vi "StopSpecificModules.vi"(8 "ErrorArray 2":errorcluster[](array[cluster]), 9 "ModuleList":string[](array[string]), 10 "ModuleIDs":i32[](array[numeric])=[-1, -1, -1], 11 "Test.lvclass 2":refnum<class "Test.lvclass">) -> (0 "ErrorArray":errorcluster[](array[cluster]), 3 "Test.lvclass":refnum<class "Test.lvclass">)   [LabVIEW 2018, in "Test.lvclass"]
uses:
  Test.lvclass
  Test.lvclass/Test.ctl
  <userlib>/NIST/ModuleAdminLib/ModuleAdmin/ModuleAdmin.lvclass
  <userlib>/NIST/ModuleAdminLib/ModuleAdmin/ModuleAdmin.lvclass/ModuleAdmin.ctl
  <userlib>/NIST/ModuleAdminLib/ModuleAdmin/Accessors/Write CloneRegRef.vi
  Accessors/Read CloneReg.vi
  <vilib>/Utility/error.llb/Error Cluster From Error Code.vi
  <userlib>/NIST/ModuleAdminLib/CloneRegistration/CloneRegistration.lvclass
  <vilib>/ErrorRing/Error Ring.xnode
  Sync/SyncModule/SyncModule.lvlib
  <userlib>/NIST/NISTErrorLib/NISTErrorLib.lvlib
  FGen/FgenModule/FgenModule.lvlib
  Digitizer/DigitizerShared/DigitizerShared.lvlib
  Scope/ScopeModule/ScopeModule.lvlib
  Sensor/SensorShared/SensorShared.lvlib
  Analysis/AnalysisModule/AnalysisModule.lvlib
  AcPwr/AcPwrModule/AcPwrModule.lvlib
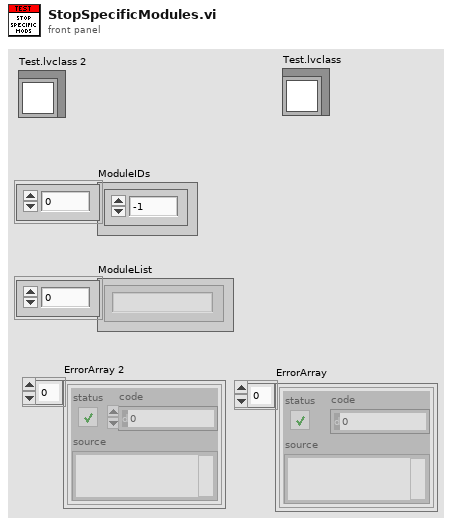
[diagram p1: front panel]
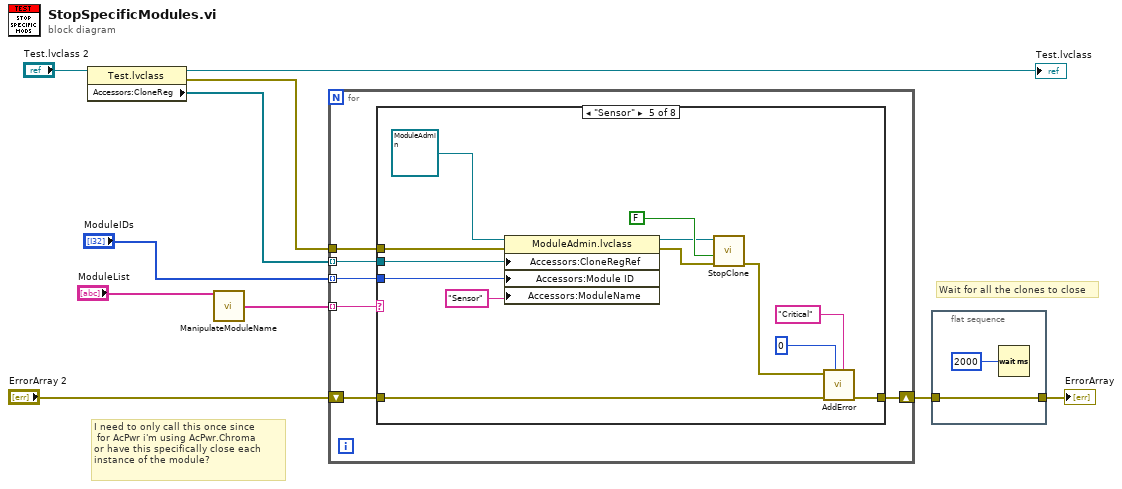
[diagram p0: block diagram]
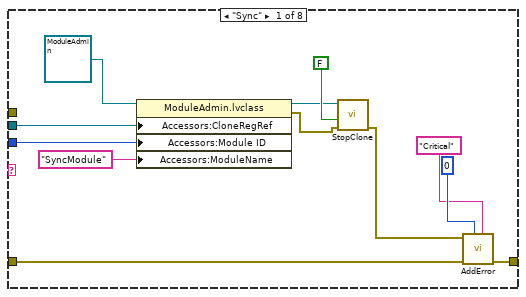
[diagram p2: hidden frame]
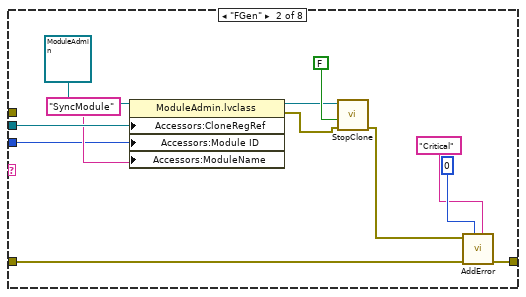
[diagram p3: hidden frame]
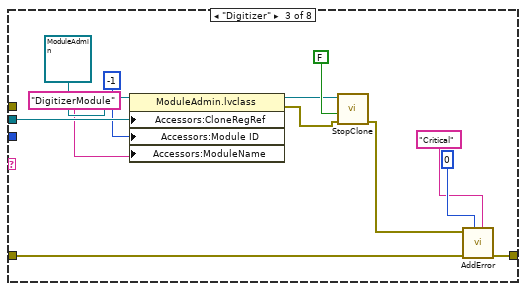
[diagram p4: hidden frame]
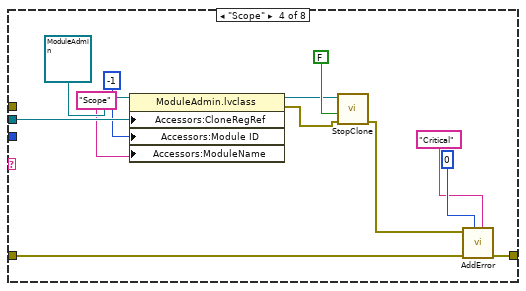
[diagram p5: hidden frame]
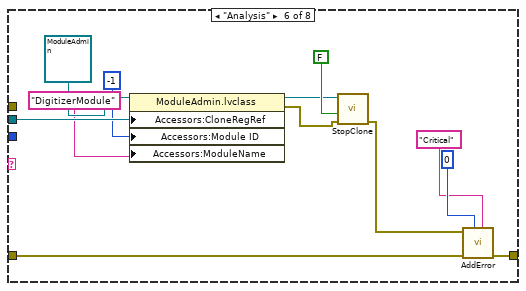
[diagram p6: hidden frame]
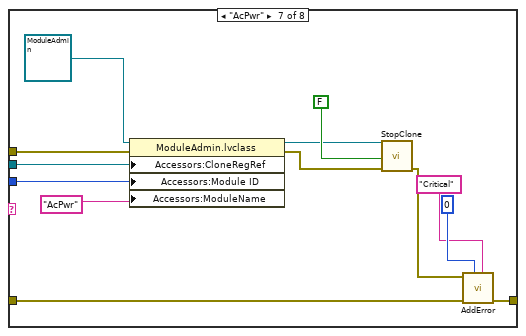
[diagram p7: hidden frame]
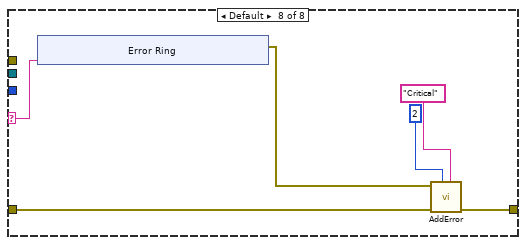
[diagram p8: hidden frame]
diagram:
  # "I need to only call this once since\n for AcPwr i'm using AcPwr.Chroma\nor have this specifically close each \ninstance of the module?"
  # "Wait for all the clones to close"
  n1 = property class="Test.lvclass"(reference="Test.lvclass 2") -> (reference out=→"Test.lvclass":refnum<class "Test.lvclass">, error out=w3:errorcluster, "Accessors:CloneReg"=w8:refnum<data-value>[])  [unwired: 1 in]
  n2 = call "ManipulateModuleName.vi"("ModuleListArrayIn"="ModuleList") -> ("BeforeMatchWithoutRedundantEntries:ModuleListArray"=w4:string[])  [unwired: 9 in, 5 out]
  n3 = for {
    shift-right: [w14] -> w6
    shift-left: "ErrorArray 2" -> [w16]
    tunnel: w8 -> [w15] mode=indexing
    tunnel: "ModuleIDs" -> [w13] mode=indexing
    tunnel: w4 -> [w12] mode=indexing
    tunnel: w3 -> [w11]
    n4 = case shown="\"Sensor\"" w12 {
      selector: w12 -> [_ _ _ _ _ _ _ w108]
      tunnel: w16 -> [w18 w30 w41 w53 w67 w78 w95 w104]
      tunnel: [w22 w34 w45 w57 w71 w82 w98 w103] -> w14
      tunnel: w15 -> [w27 w39 w51 w63 w76 w88 w101 _]
      tunnel: w13 -> [w17 w29 _ _ w65 _ w91 _]
      tunnel: w11 -> [_ _ _ _ w66 _ w90 _]
      frame "Sync" {
        n5 = property class="ModuleAdmin.lvclass"(reference=refnum<class "ModuleAdmin.lvclass"> refnum ("ModuleAdmin.lvlib:ModuleAdmin.lvclass"), "Accessors:CloneRegRef"=w27, "Accessors:Module ID"=w17, "Accessors:ModuleName"="SyncModule" ("ModuleName")) -> (reference out=w24:refnum<class "ModuleAdmin.lvclass">, error out=w23:errorcluster)  [unwired: 1 in]
        n6 = call "StopClone.vi"("error in (no error)"=w23, "Wait for Module to stop?"=FALSE, "ModuleAdmin"=w24) -> ("error out"=w19:errorcluster)  [unwired: 8 in]
        n7 = call <userlib>:"AddError.vi"("Severity"="Critical", "Priority"=u8 0, "ErrorArray"=w18, "error in (no error)"=w19) -> ("ErrorArray"=w22:errorcluster[])  [unwired: 6 in, 1 out]
      }
      frame "FGen" {
        n8 = property class="ModuleAdmin.lvclass"(reference=refnum<class "ModuleAdmin.lvclass"> refnum ("ModuleAdmin.lvlib:ModuleAdmin.lvclass"), "Accessors:CloneRegRef"=w39, "Accessors:Module ID"=w29, "Accessors:ModuleName"="SyncModule" ("ModuleName")) -> (reference out=w36:refnum<class "ModuleAdmin.lvclass">, error out=w35:errorcluster)  [unwired: 1 in]
        n9 = call "StopClone.vi"("error in (no error)"=w35, "Wait for Module to stop?"=FALSE, "ModuleAdmin"=w36) -> ("error out"=w31:errorcluster)  [unwired: 8 in]
        n10 = call <userlib>:"AddError.vi"("Severity"="Critical", "Priority"=u8 0, "ErrorArray"=w30, "error in (no error)"=w31) -> ("ErrorArray"=w34:errorcluster[])  [unwired: 6 in, 1 out]
      }
      frame "Digitizer" {
        n11 = property class="ModuleAdmin.lvclass"(reference=refnum<class "ModuleAdmin.lvclass"> refnum ("ModuleAdmin.lvlib:ModuleAdmin.lvclass"), "Accessors:CloneRegRef"=w51, "Accessors:Module ID"=-1 ("Module ID"), "Accessors:ModuleName"="DigitizerModule" ("ModuleName")) -> (reference out=w47:refnum<class "ModuleAdmin.lvclass">, error out=w46:errorcluster)  [unwired: 1 in]
        n12 = call "StopClone.vi"("error in (no error)"=w46, "Wait for Module to stop?"=FALSE, "ModuleAdmin"=w47) -> ("error out"=w42:errorcluster)  [unwired: 8 in]
        n13 = call <userlib>:"AddError.vi"("Severity"="Critical", "Priority"=u8 0, "ErrorArray"=w41, "error in (no error)"=w42) -> ("ErrorArray"=w45:errorcluster[])  [unwired: 6 in, 1 out]
      }
      frame "Scope" {
        n14 = property class="ModuleAdmin.lvclass"(reference=refnum<class "ModuleAdmin.lvclass"> refnum ("ModuleAdmin.lvlib:ModuleAdmin.lvclass"), "Accessors:CloneRegRef"=w63, "Accessors:Module ID"=-1 ("Module ID"), "Accessors:ModuleName"="Scope" ("ModuleName")) -> (reference out=w59:refnum<class "ModuleAdmin.lvclass">, error out=w58:errorcluster)  [unwired: 1 in]
        n15 = call "StopClone.vi"("error in (no error)"=w58, "Wait for Module to stop?"=FALSE, "ModuleAdmin"=w59) -> ("error out"=w54:errorcluster)  [unwired: 8 in]
        n16 = call <userlib>:"AddError.vi"("Severity"="Critical", "Priority"=u8 0, "ErrorArray"=w53, "error in (no error)"=w54) -> ("ErrorArray"=w57:errorcluster[])  [unwired: 6 in, 1 out]
      }
      frame "Sensor" {
        n17 = property class="ModuleAdmin.lvclass"(reference=refnum<class "ModuleAdmin.lvclass"> refnum ("ModuleAdmin.lvlib:ModuleAdmin.lvclass"), error in=w66, "Accessors:CloneRegRef"=w76, "Accessors:Module ID"=w65, "Accessors:ModuleName"="Sensor" ("ModuleName")) -> (reference out=w73:refnum<class "ModuleAdmin.lvclass">, error out=w72:errorcluster)
        n18 = call "StopClone.vi"("error in (no error)"=w72, "Wait for Module to stop?"=FALSE, "ModuleAdmin"=w73) -> ("error out"=w68:errorcluster)  [unwired: 8 in]
        n19 = call <userlib>:"AddError.vi"("Severity"="Critical", "Priority"=u8 0, "ErrorArray"=w67, "error in (no error)"=w68) -> ("ErrorArray"=w71:errorcluster[])  [unwired: 6 in, 1 out]
      }
      frame "Analysis" {
        n20 = property class="ModuleAdmin.lvclass"(reference=refnum<class "ModuleAdmin.lvclass"> refnum ("ModuleAdmin.lvlib:ModuleAdmin.lvclass"), "Accessors:CloneRegRef"=w88, "Accessors:Module ID"=-1 ("Module ID"), "Accessors:ModuleName"="DigitizerModule" ("ModuleName")) -> (reference out=w84:refnum<class "ModuleAdmin.lvclass">, error out=w83:errorcluster)  [unwired: 1 in]
        n21 = call "StopClone.vi"("error in (no error)"=w83, "Wait for Module to stop?"=FALSE, "ModuleAdmin"=w84) -> ("error out"=w79:errorcluster)  [unwired: 8 in]
        n22 = call <userlib>:"AddError.vi"("Severity"="Critical", "Priority"=u8 0, "ErrorArray"=w78, "error in (no error)"=w79) -> ("ErrorArray"=w82:errorcluster[])  [unwired: 6 in, 1 out]
      }
      frame "AcPwr" {
        n23 = property class="ModuleAdmin.lvclass"(reference=refnum<class "ModuleAdmin.lvclass"> refnum ("ModuleAdmin.lvlib:ModuleAdmin.lvclass"), error in=w90, "Accessors:CloneRegRef"=w101, "Accessors:Module ID"=w91, "Accessors:ModuleName"="AcPwr" ("ModuleName")) -> (reference out=w92:refnum<class "ModuleAdmin.lvclass">, error out=w99:errorcluster)
        n24 = call "StopClone.vi"("error in (no error)"=w99, "Wait for Module to stop?"=FALSE, "ModuleAdmin"=w92) -> ("error out"=w94:errorcluster)  [unwired: 8 in]
        n25 = call <userlib>:"AddError.vi"("Severity"="Critical", "Priority"=u8 0, "ErrorArray"=w95, "error in (no error)"=w94) -> ("ErrorArray"=w98:errorcluster[])  [unwired: 6 in, 1 out]
      }
      frame Default {
        n26 = xnode "Error Ring"("parameter 0"=w108) -> ("error out"=w105:errorcluster)
        n27 = call <userlib>:"AddError.vi"("Severity"="Critical", "Priority"=u8 2, "ErrorArray"=w104, "error in (no error)"=w105) -> ("ErrorArray"=w103:errorcluster[])  [unwired: 6 in, 1 out]
      }
    }
  }
  n28 = flat-sequence {
    tunnel: [w117] -> w5
    tunnel: w6 -> [w117]
    frame #0 {
      n29 = Wait (ms)(milliseconds to wait=u32 2000) -> ()  [unwired: 1 out]
    }
  }
  "ErrorArray" <- w5
